vi "FeedbackDecode_WriteVideoParams.vi"(6 "FileTime":string, 8 "ErrorIn":errorcluster, 9 "DataPath":path=path "D:/00000000-000000", 10 "Frame":string="-1", 11 "Mode":enum16{"Initialize", "Run", "Close"}(ring)) -> (0 "ErrorOut":errorcluster, 2 "VideoParamsName":path)   [LabVIEW 2020]
uses:
  FeedbackDecode_Globals.vi
panel:
  out "VideoParamsFID":refnum<file>
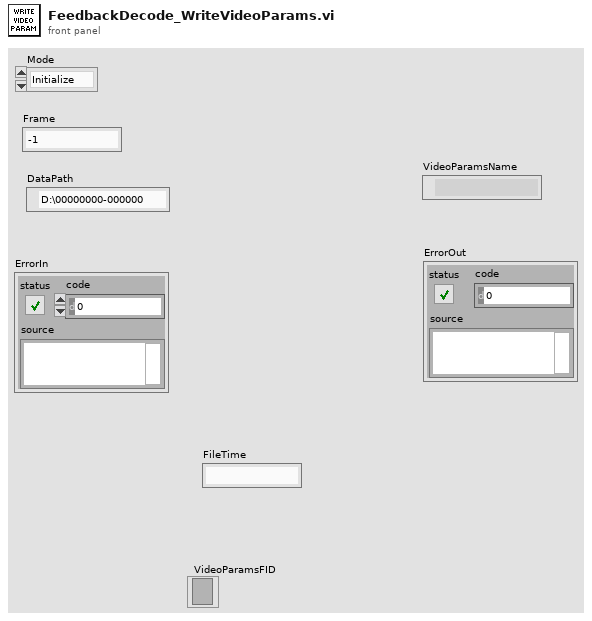
[diagram p1: front panel]
types:
  T1 = enum16{"open", "replace", "create", "open or create", "replace or create", "replace or create with confirmation"}
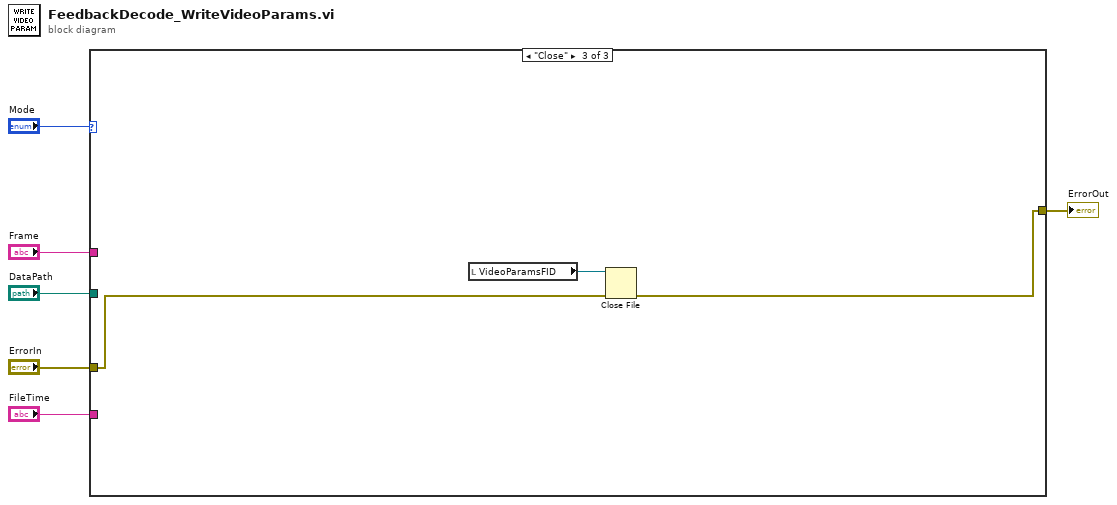
[diagram p0: block diagram]
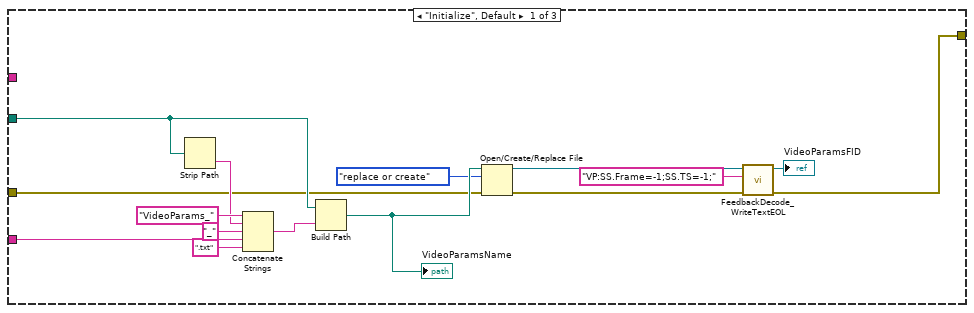
[diagram p2: hidden frame]
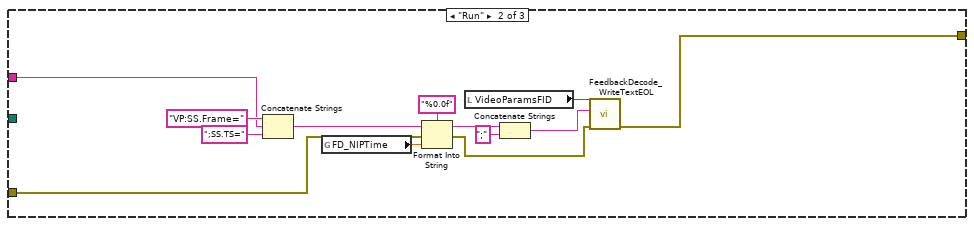
[diagram p3: hidden frame]
diagram:
  n1 = case shown="\"Close\"" "Mode" {
    tunnel: "ErrorIn" -> [w11 w23 w36]
    tunnel: [w14 w25 w35] -> w4
    tunnel: "DataPath" -> [w12 _ _]
    tunnel: "Frame" -> [_ w24 _]
    tunnel: "FileTime" -> [w8 _ _]
    frame "Initialize", Default {
      n2 = Strip Path(path=w12) -> (name=w16:string)  [unwired: 1 out]
      n3 = Concatenate Strings("VideoParams_" ("name or relative path"), w16, "_" ("string"), w8, ".txt" ("string")) -> (w17:string)
      n4 = Build Path(base path=w12, name or relative path=w17) -> (appended path=w21:path)
      "VideoParamsName" <- w21
      n5 = Open/Create/Replace File(file path (use dialog)=w21, error in=w11, operation (0:open)=T1."replace or create") -> (refnum out=w15:refnum<file>, error out=w9:errorcluster)  [unwired: 3 in, 1 out]
      n6 = call "FeedbackDecode_WriteTextEOL.vi"("error in"=w9, "text"="VP:SS.Frame=-1;SS.TS=-1;" ("string"), "refnum in"=w15) -> ("error out"=w14:errorcluster, "refnum out"=→"VideoParamsFID":refnum<file>)  [unwired: 7 in]
    }
    frame "Run" {
      n7 = Concatenate Strings("VP:SS.Frame=" ("string"), w24, ";SS.TS=" ("string")) -> (w28:string)
      n8 = global read "FeedbackDecode_Globals.vi" "FD_NIPTime"() -> (w22:dbl)
      n9 = Format Into String(format string="%0.0f", initial string=w28, error in=w23, w22) -> (resulting string=w30:string, error out=w26:errorcluster)
      n10 = local read "VideoParamsFID"() -> (w34:refnum<file>)
      n11 = Concatenate Strings(w30, ";" ("string")) -> (w27:string)
      n12 = call "FeedbackDecode_WriteTextEOL.vi"("error in"=w26, "text"=w27, "refnum in"=w34) -> ("error out"=w25:errorcluster)  [unwired: 7 in, 1 out]
    }
    frame "Close" {
      n13 = local read "VideoParamsFID"() -> (w37:refnum<file>)
      n14 = Close File(refnum=w37, error in=w36) -> (error out=w35:errorcluster)  [unwired: 1 out]
    }
  }
  "ErrorOut" <- w4
